vi "topic.get.vi"(8 "error in (no error)":errorcluster, 11 "topic in":refnum<class "topic.lvclass">) -> (0 "error out":errorcluster, 2 "topic":string, 3 "topic out":refnum<class "topic.lvclass">)   [LabVIEW 2020, in "nominal types.lvlib" / "channelFilter.lvlib" / "topic.lvclass"]
uses:
  topic.lvclass
  topic.lvclass/topic.ctl
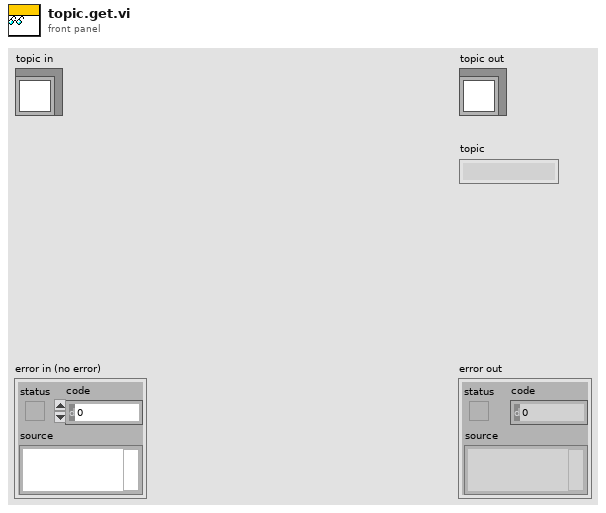
[diagram p1: front panel]
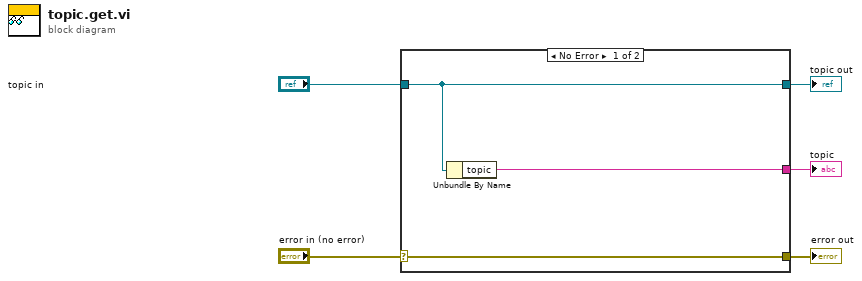
[diagram p0: block diagram]
diagram:
  n1 = case shown="No Error" "error in (no error)" {
    selector: "error in (no error)" -> [w8 w9]
    tunnel: [w8 w9] -> w4
    tunnel: [w7 w10] -> w2
    tunnel: "topic in" -> [w7 w10]
    tunnel: [w6 _] -> w1
    frame No Error {
      n2 = Unbundle By Name(w7) -> ("topic"=w6:string)
    }
    frame Error {
    }
  }
  "error out" <- w4
  "topic out" <- w2
  "topic" <- w1
